vi "ParseSaveFile.vi"(8 "error in (no error)":errorcluster, 11 "ExpData File Path":path) -> (0 "error out":errorcluster, 1 "Data":string[][](array[string]), 2 "MetaData":string, 3 "dup path":path, 4 "Column Headers":string[](array[string]))   [LabVIEW 2016, in "ExpData.lvclass"]
uses:
  ExpData.lvclass
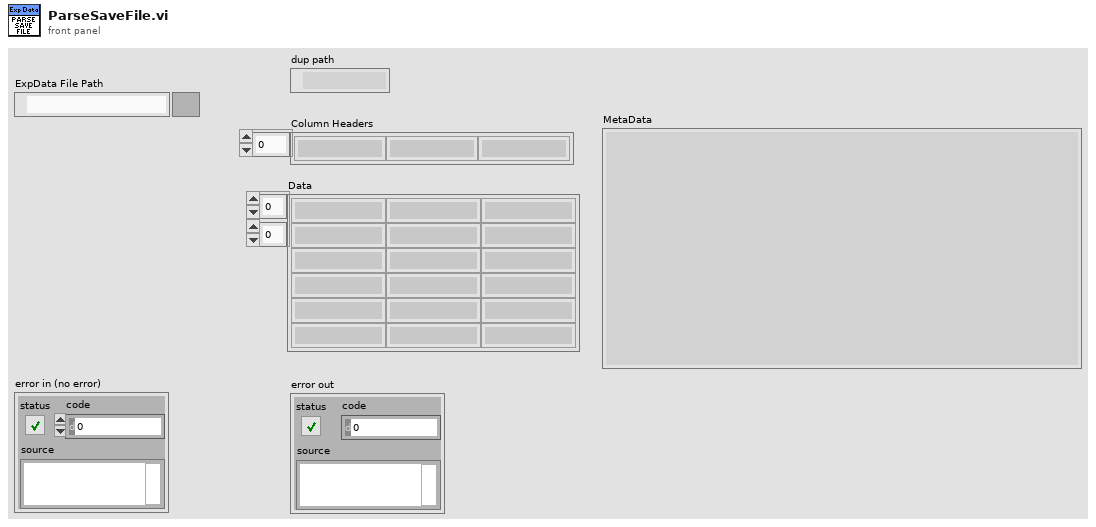
[diagram p1: front panel]
types:
  T1 = enum16{"Native", "Native Command Line", "UNIX", "Macintosh", "DOS"}
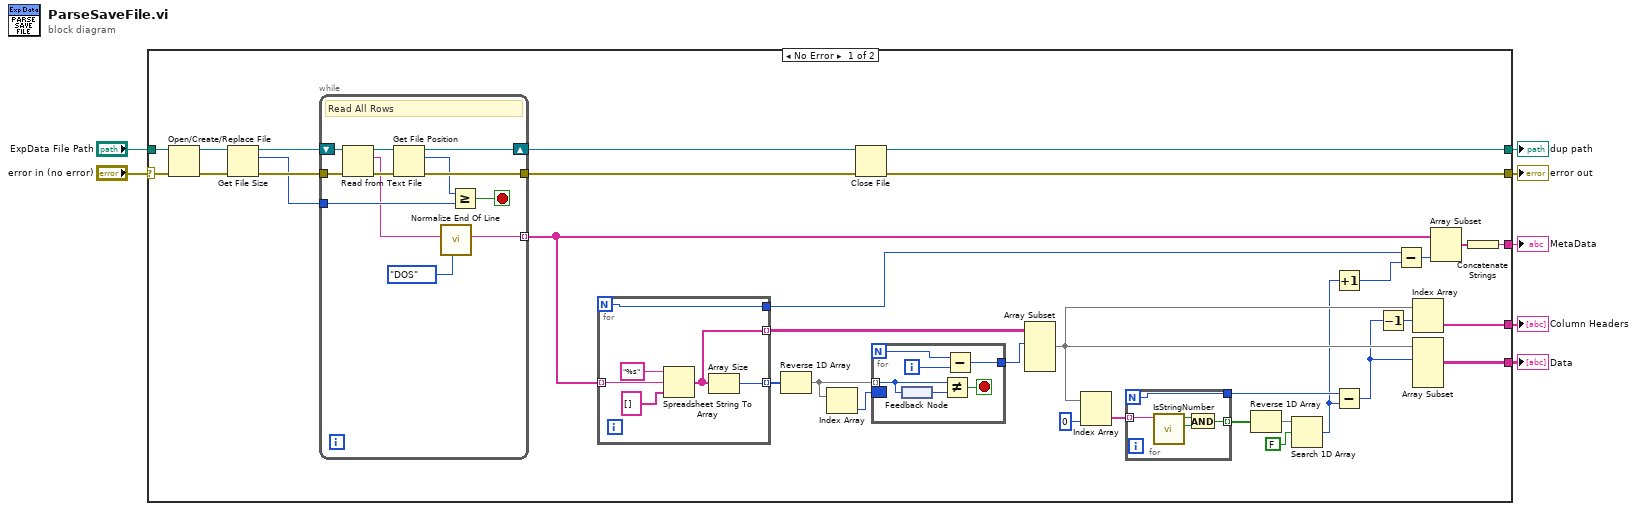
[diagram p0: block diagram]
diagram:
  n1 = case shown="No Error" "error in (no error)" {
    selector: "error in (no error)" -> [w8 w71]
    tunnel: [w41 w71] -> w7
    tunnel: [w40 w72] -> w6
    tunnel: "ExpData File Path" -> [w39 w72]
    tunnel: [w22 _] -> w4
    tunnel: [w19 _] -> w3
    tunnel: [w11 _] -> w2
    frame No Error {
      n2 = Open/Create/Replace File(file path (use dialog)=w39, error in=w8) -> (refnum out=w36:refnum<file>, error out=w34:errorcluster)  [unwired: 4 in, 1 out]
      n3 = Get File Size(file=w36, error in=w34) -> (refnum out=w35:refnum<file>, size (in bytes)=w32:i64, 0:w33:errorcluster)
      n4 = while {
        tunnel: w33 -> [w69]
        tunnel: [w66] -> w38
        shift-right: [w65] -> w37
        shift-left: w35 -> [w70]
        tunnel: [w60] -> w18 mode=indexing
        tunnel: w32 -> [w63]
        stop <- w62 stop-if-true
        # "Read All Rows"
        n5 = Read from Text File(file (use dialog)=w70, error in=w69) -> (refnum out=w68:refnum<file>, text=w61:string, error out=w67:errorcluster)  [unwired: 2 in, 1 out]
        n6 = Get File Position(4:w67, 7:w68) -> (0:w66:errorcluster, 2:w64:i64, 3:w65:refnum<file>)
        n7 = call <vilib>:"Normalize End Of Line.vi"("end of line (Native)"=T1."DOS", "string in"=w61) -> ("string out"=w60:string)  [unwired: 6 in]
        n8 = Greater Or Equal?(x=w64, y=w63) -> (x >= y?=w62:bool)
      }
      n9 = for {
        N -> [w53]
        tunnel: w18 -> [w58] mode=indexing
        tunnel: [w55] -> w30 mode=indexing
        tunnel: [w54] -> w31 mode=indexing
        tunnel: [w53] -> w15
        n10 = Spreadsheet String To Array(format string="%s", spreadsheet string=w58, array type (2D Dbl)=string[] []) -> (array=w55:string[])  [unwired: 1 in]
        n11 = Array Size(array=w55) -> (size(s)=w54:i32)
      }
      n12 = Reverse 1D Array(array=w31) -> (reversed array=w10:i32[])
      n13 = Index Array(array=w10) -> (element=w9:i32)  [unwired: 1 in]
      n14 = Close File(refnum=w37, error in=w38) -> (path=w40:path, error out=w41:errorcluster)
      n15 = for {
        N -> [w48]
        tunnel: w10 -> [w51] mode=indexing
        tunnel: [w47] -> w29
        border: w9 -> [_]
        i -> [w49]
        stop <- w50 stop-if-true
        n16 = feedback #1() -> (w52:i32)
        n17 = feedback-in #1(w51) -> ()
        n18 = Not Equal?(x=w51, y=w52) -> (x != y?=w50:bool)
        n19 = Subtract(x=w48, y=w49) -> (x-y=w47:i32)
      }
      n20 = Array Subset(array=w30, index (row)=w29) -> (w21:string[][])  [unwired: 3 in]
      n21 = Index Array(array=w21, index (col)=0 ("disabled index (col)")) -> (element=w28:string[])  [unwired: 1 in]
      n22 = for {
        N -> [w42]
        tunnel: w28 -> [w43] mode=indexing
        tunnel: [w44] -> w26 mode=indexing
        tunnel: [w42] -> w23
        n23 = call "IsStringNumber.vi"("String"=w43) -> ("End with Number"=w45:bool, "Start with Number"=w46:bool)  [unwired: 7 in, 2 out]
        n24 = And(x=w46, y=w45) -> (x .and. y?=w44:bool)
      }
      n25 = Reverse 1D Array(array=w26) -> (reversed array=w25:bool[])
      n26 = Search 1D Array(1D array=w25, element=FALSE) -> (index of element=w14:i32)  [unwired: 1 in]
      n27 = Increment(x=w14) -> (x+1=w13:i32)
      n28 = Subtract(x=w23, y=w14) -> (x-y=w16:i32)
      n29 = Decrement(x=w16) -> (x-1=w20:i32)
      n30 = Subtract(x=w15, y=w13) -> (x-y=w17:i32)
      n31 = Index Array(array=w21, index (row)=w20) -> (element=w19:string[])  [unwired: 1 in]
      n32 = Array Subset(array=w21, index (row)=w16) -> (w22:string[][])  [unwired: 3 in]
      n33 = Array Subset(array=w18, length=w17) -> (w12:string[])  [unwired: 1 in]
      n34 = Concatenate Strings(w12) -> (w11:string)
    }
    frame Error {
    }
  }
  "MetaData" <- w2
  "error out" <- w7
  "dup path" <- w6
  "Column Headers" <- w3
  "Data" <- w4
